vi "imagine to array.vi"(11 "image data":T1) -> (0 "array imagine":dbl[](array[numeric]), 3 "Intensity Graph":dbl[][](graph))   [LabVIEW 2024]
uses:
  <vilib>/picture/picture.llb/imagedata.ctl
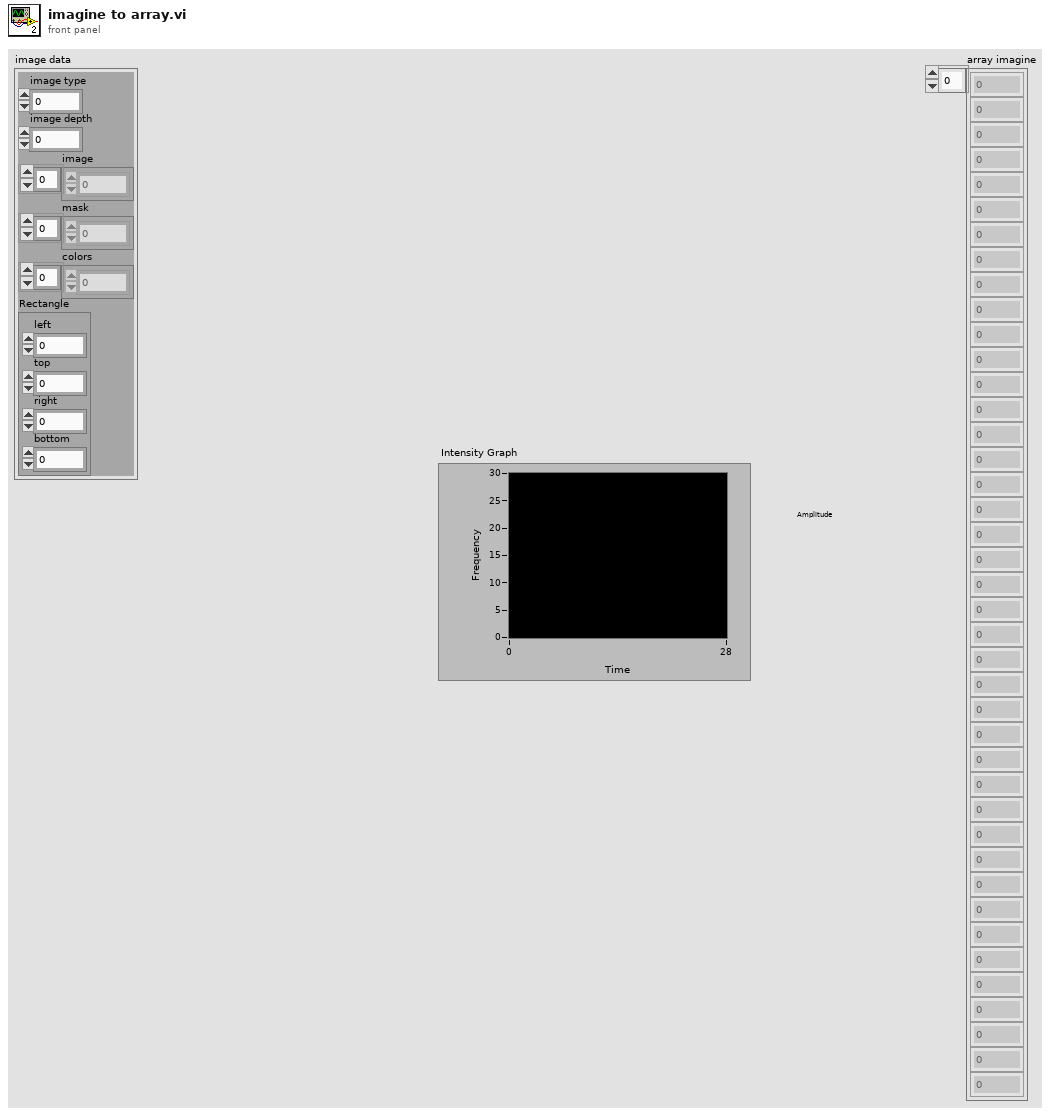
[diagram p1: front panel]
types:
  T1 = typedef "imagedata.ctl" = cluster{"image type":i32, "image depth":i32, "image":u8[], "mask":u8[], "colors":u32[], "Rectangle":cluster{"left":i16, "top":i16, "right":i16, "bottom":i16}}
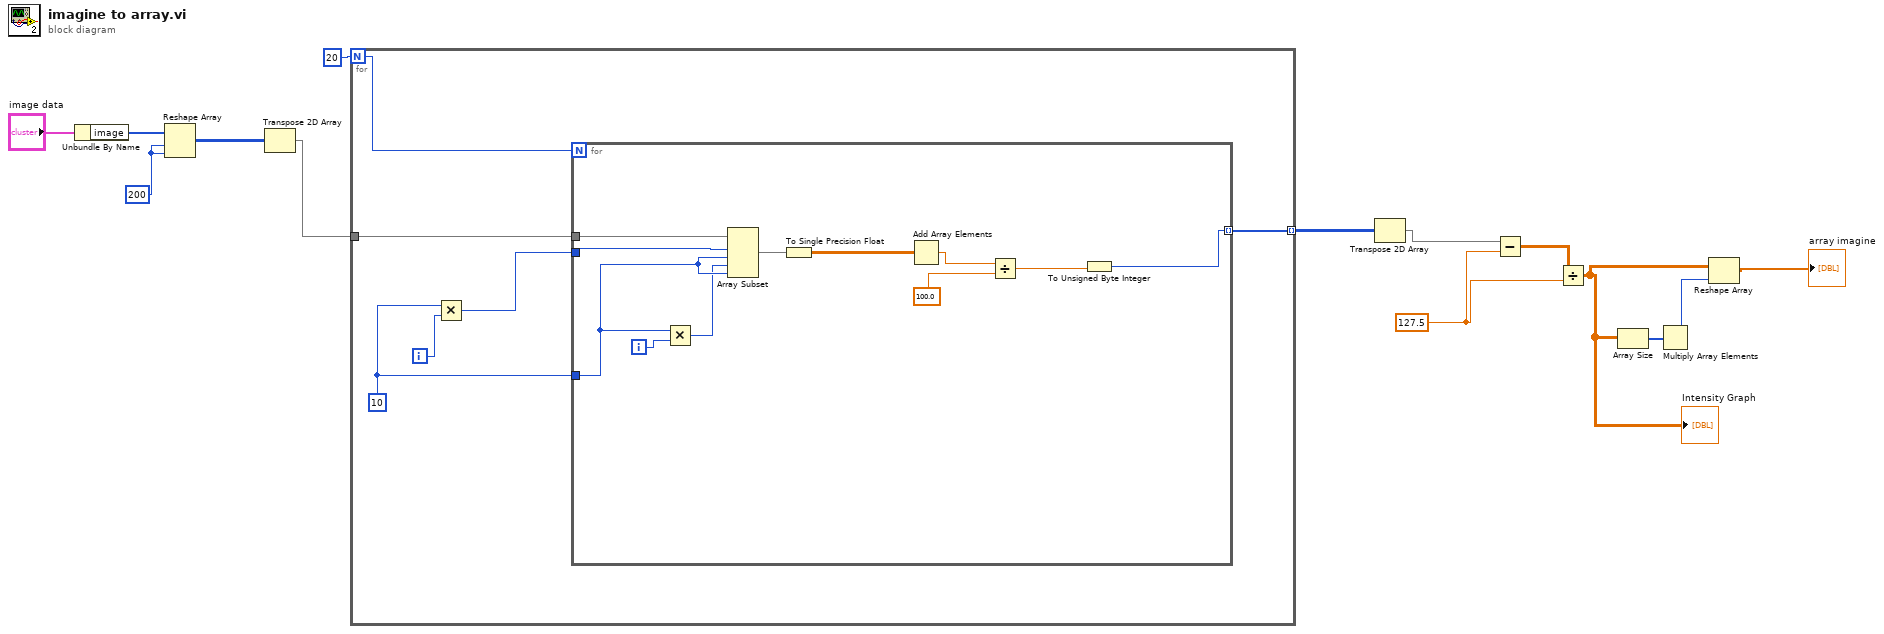
[diagram p0: block diagram]
diagram:
  w6 = 127.5
  w13 = 200
  n1 = Unbundle By Name("image data") -> ("image"=w14:u8[])
  n2 = Reshape Array "Reshape Array"(w14, w13, w13) -> (w12:u8[][])
  n3 = Transpose 2D Array(2D array=w12) -> (transposed array=w10:u8[][])
  n4 = for {
    N: 20 -> [w20]
    tunnel: w10 -> [w18]
    tunnel: [w15] -> w9 mode=indexing
    i -> [w19]
    w16 = 10 ("x")
    n5 = Multiply(x=w16, y=w19) -> (x*y=w17:i32)
    n6 = for {
      N: w20 -> [_]
      tunnel: w18 -> [w31]
      tunnel: w17 -> [w30]
      tunnel: w16 -> [w28]
      tunnel: [w21] -> w15 mode=indexing
      i -> [w29]
      n7 = Multiply(x=w28, y=w29) -> (x*y=w27:i32)
      n8 = Array Subset "Array Subset"(array=w31, index (row)=w30, length (row)=w28, index (col)=w27, length (col)=w28) -> (w26:u8[][])
      n9 = To Single Precision Float(number=w26) -> (single precision float=w24:sgl[][])
      n10 = Add Array Elements(numeric array=w24) -> (sum=w23:sgl)
      n11 = Divide(x=w23, y=sgl 100.0) -> (x/y=w22:sgl)
      n12 = To Unsigned Byte Integer(number=w22) -> (unsigned 8bit integer=w21:u8)
    }
  }
  n13 = Transpose 2D Array(2D array=w9) -> (transposed array=w8:u8[][])
  n14 = Subtract(x=w8, y=w6) -> (x-y=w7:dbl[][])
  n15 = Divide(x=w7, y=w6) -> (x/y=w2:dbl[][])
  "Intensity Graph" <- w2
  n16 = Array Size(array=w2) -> (size(s)=w5:i32[])
  n17 = Multiply Array Elements(1:w5) -> (0:w4:i32)
  n18 = Reshape Array "Reshape Array"(w2, w4) -> (→"array imagine":dbl[])
